vi "readFromXMLAzElParameters.vi"(8 "error in (no error)":errorcluster, 10 "XMLin":string="<AzElParameters>\n  <azimuth>\n    <degreesArc>44.44</degreesArc>\n    <minutesArc>33.33</minutesArc>\n    <secondsArc>22.22</secondsArc>\n  </azimuth>\n  <elevation>\n    <degreesAlt>90.20</degreesAlt>\n    <minutesArc>80.30</minutesArc>\n    <secondsArc>70.40</secondsArc>\n  </elevation>\n</AzElParameters>") -> (0 "error out":errorcluster)   [LabVIEW 2012]
uses:
  <userlib>/Common/XML/XMLParser/XMLParser.lvclass
  <userlib>/Common/XML/Typedefs/AttributeElements.ctl
  <userlib>/Common/XML/XML.lvlib
panel:
  out "childAttributes":T1[](array[typedef])
  out "Element out":refnum<class "XMLParser.lvclass">
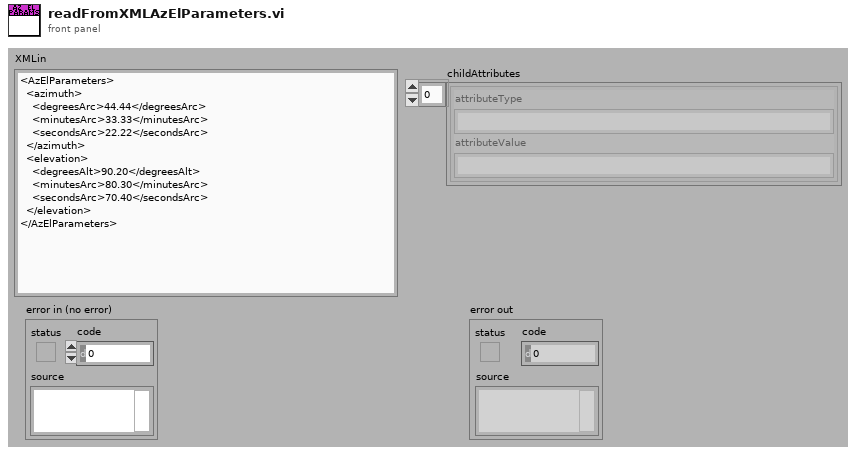
[diagram p1: front panel]
types:
  T1 = typedef "XML.lvlib/AttributeElements.ctl" = cluster{"attributeType":string, "attributeValue":string}
  T2 = typedef "AttributeElements.ctl" = cluster{"attributeType":string, "attributeValue":string}
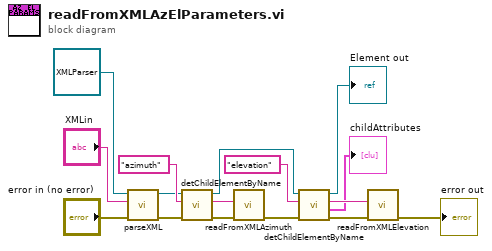
[diagram p0: block diagram]
diagram:
  n1 = call <userlib>:"parseXML.vi"("error in (no error)"="error in (no error)", "XMLString in"="XMLin", "Element in"=refnum<class "XMLParser.lvclass"> refnum) -> ("error out"=w10:errorcluster, "Element out"=w11:refnum<class "XMLParser.lvclass">)  [unwired: 7 in]
  n2 = call <userlib>:"detChildElementByName.vi"("error in (no error)"=w10, "childName"="azimuth" ("ChildName"), "Element in"=w11) -> ("error out"=w3:errorcluster, "childXML"=w9:string, "Element out"=w6:refnum<class "XMLParser.lvclass">)  [unwired: 5 in, 1 out]
  n3 = call <userlib>:"readFromXMLAzimuth.vi"("error in (no error)"=w3, "XML in"=w9) -> ("error out"=w7:errorcluster)  [unwired: 9 in]
  n4 = call <userlib>:"detChildElementByName.vi"("error in (no error)"=w7, "childName"="elevation" ("ChildName"), "Element in"=w6) -> ("error out"=w4:errorcluster, "childAttributes"=→"childAttributes":T2[], "childXML"=w5:string, "Element out"=→"Element out":refnum<class "XMLParser.lvclass">)  [unwired: 5 in]
  n5 = call <userlib>:"readFromXMLElevation.vi"("error in (no error)"=w4, "XML in"=w5) -> ("error out"=→"error out":errorcluster)  [unwired: 9 in]
